vi "串口配置.vi"(11 "VISA资源名称":refnum<visa-resource-name>) -> (2 "确认 2":bool, 3 "VISA资源名称 2":refnum<visa-resource-name>)   [LabVIEW 2016, in "斯坦道CODMn.lvlib"]
panel:
  in  "取消":bool
  in  "确认":bool
  # "请选择串口:"
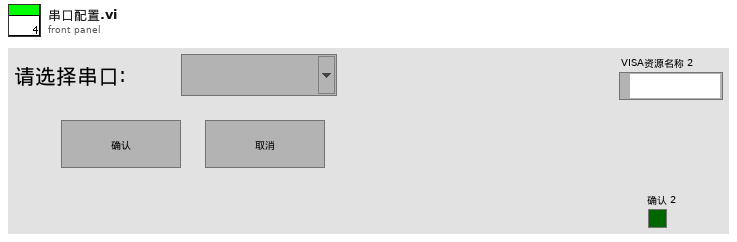
[diagram p1: front panel]
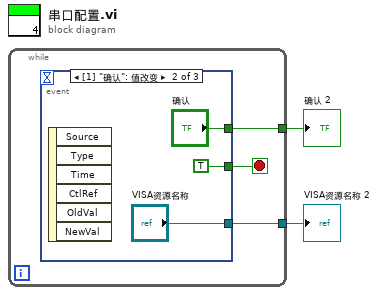
[diagram p0: block diagram]
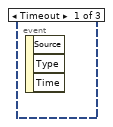
[diagram p2: hidden frame]
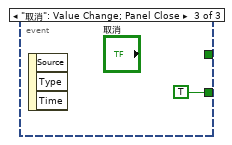
[diagram p3: hidden frame]
diagram:
  n1 = while {
    tunnel: [w5] -> w2
    tunnel: [w3] -> w1
    stop <- w4 stop-if-true
    n2 = event shown="[1] \"确认\": 值改变" {
      selector: _ -> [_ _ _]
      dyn-events: _ -> [_ _ _]
      timeout: _ -> [_ _ _]
      tunnel: [_ "VISA资源名称" _] -> w5
      tunnel: [_ TRUE TRUE] -> w4
      tunnel: [_ "确认" _] -> w3
      event Timeout {
        n3 = event-data() -> ()  [unwired: 1 in, 3 out]
      }
      event "确认": Value Change {
        n4 = event-data() -> ()  [unwired: 1 in, 6 out]
      }
      event "取消": Value Change; Panel Close {
        n5 = event-data() -> ()  [unwired: 1 in, 3 out]
      }
    }
  }
  "VISA资源名称 2" <- w2
  "确认 2" <- w1
